vi "fpga_next_position_1ch.vi"(7 "speed":sgl, 10 "ready to move?":bool, 11 "target":sgl) -> (2 "move completed?":bool, 3 "output (out)":sgl)   [LabVIEW 2021]
doc: "This is a sub vi to calculate the next position.\n\nThis vi calculate a next position of single channel. The current position is stored in this vi."
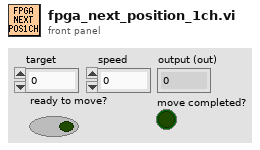
[diagram p1: front panel]
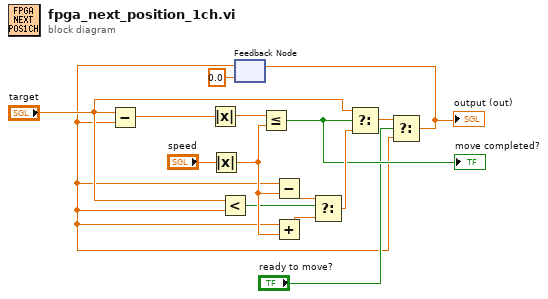
[diagram p0: block diagram]
diagram:
  n1 = Absolute Value(x="speed") -> (abs(x)=w14:sgl)
  n2 = feedback #1(sgl 0.0 ("target")) -> (w3:sgl)
  n3 = Subtract(x="target", y=w3) -> (x-y=w13:sgl)
  n4 = Absolute Value(x=w13) -> (abs(x)=w1:sgl)
  n5 = Less?(x="target", y=w3) -> (x < y?=w2:bool)
  n6 = Less Or Equal?(x=w1, y=w14) -> (x <= y?=w9:bool)
  "move completed?" <- w9
  n7 = Subtract(x=w3, y=w14) -> (x-y=w12:sgl)
  n8 = Add(x=w3, y=w14) -> (x+y=w11:sgl)
  n9 = Select(t=w12, s=w2, f=w11) -> (s? t:f=w10:sgl)
  n10 = Select(t="target", s=w9, f=w10) -> (s? t:f=w7:sgl)
  n11 = Select(t=w7, s="ready to move?", f=w3) -> (s? t:f=w5:sgl)
  "output (out)" <- w5
  n12 = feedback-in #1(w5) -> ()
